vi "Launch WriteUR Core.vi"(8 "error in":errorcluster, 11 "Master CR":refnum<class "WebSocket Client CR.lvclass">) -> (0 "error out":errorcluster)   [LabVIEW 2021]
uses:
  WebSocket Client CR.lvclass
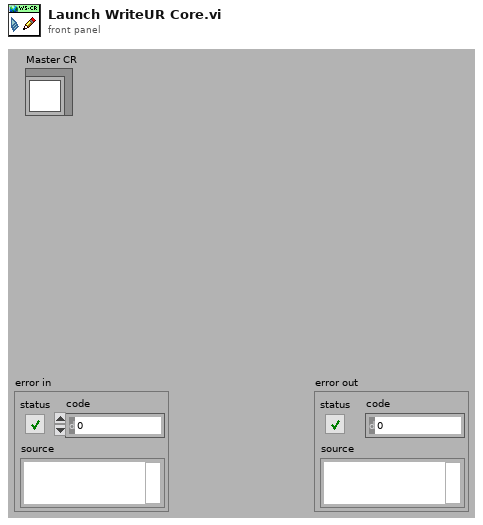
[diagram p1: front panel]
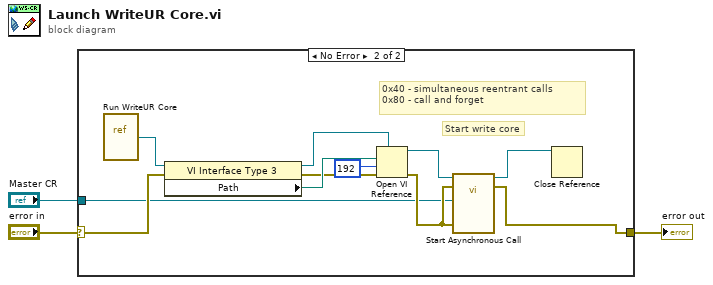
[diagram p0: block diagram]
diagram:
  n1 = case shown="No Error" "error in" {
    selector: "error in" -> [w4 w9]
    tunnel: [w4 w5] -> w3
    tunnel: "Master CR" -> [_ w6]
    frame Error {
    }
    frame No Error {
      # "Start write core"
      # "0x40 - simultaneous reentrant calls\n0x80 - call and forget"
      n2 = vi-ref "Run WriteUR Core.vi"() -> (w15:refnum<vi>)
      n3 = property class="VI Interface Type 3"(reference=w15, error in=w9) -> (reference out=w10:refnum<vi>, error out=w8:errorcluster, "Path"=w14:path)
      n4 = Open VI Reference(type specifier VI Refnum (for type only)=w10, vi path=w14, options=192, error in (no error)=w8) -> (vi reference=w13:refnum<vi>, error out=w7:errorcluster)  [unwired: 2 in]
      n5 = call-by-ref "Start Asynchronous Call"(reference=w13, error in=w7, 8:"error in (no error)"=w7, "MB in"=w6) -> (reference out=w11:refnum<vi>, error out=w5:errorcluster)  [unwired: 9 in, 1 out]
      n6 = Close Reference(reference=w11) -> ()  [unwired: 1 in, 1 out]
    }
  }
  "error out" <- w3
